vi "Read System.vi"(8 "error in (no error)":errorcluster, 11 "Master in":refnum<class "Master.lvclass">) -> (0 "error out":errorcluster, 3 "Master out":refnum<class "Master.lvclass">)   [LabVIEW 2014, in "Master.lvclass"]
uses:
  Master/Master.lvclass
  Master/Master.lvclass/Master.ctl
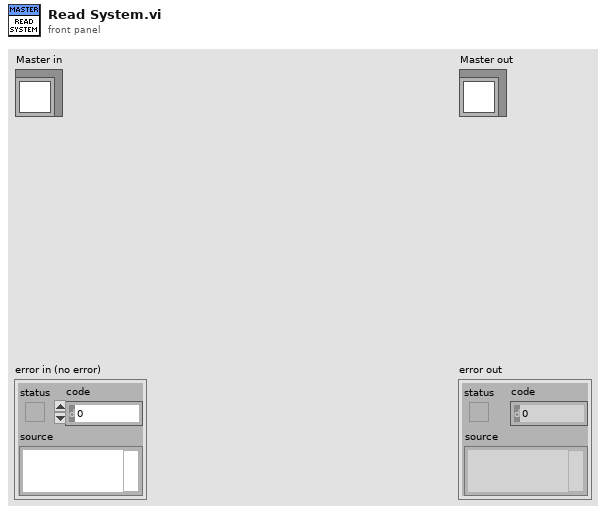
[diagram p1: front panel]
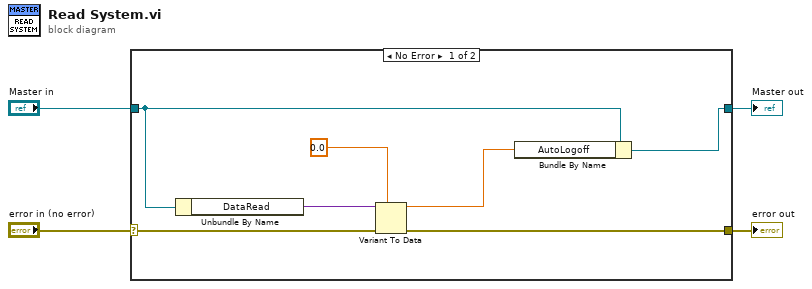
[diagram p0: block diagram]
diagram:
  n1 = case shown="No Error" "error in (no error)" {
    selector: "error in (no error)" -> [w11 w13]
    tunnel: [w10 w13] -> w3
    tunnel: [w7 w12] -> w1
    tunnel: "Master in" -> [w8 w12]
    frame No Error {
      n2 = Unbundle By Name(w8) -> ("DataRead"=w9:variant)
      n3 = Variant To Data(error in=w11, type=0.0, Variant=w9) -> (data=w6:dbl, error out=w10:errorcluster)
      n4 = Bundle By Name(cluster=w8, "AutoLogoff"=w6) -> (w7:refnum<class "Master.lvclass">)
    }
    frame Error {
    }
  }
  "error out" <- w3
  "Master out" <- w1
